vi "FindFocus.vi"(8 "error in (no error)":errorcluster, 11 "Transport":refnum<class "Transport.lvclass">) -> (0 "error out":errorcluster, 3 "Transport.lvclass":refnum<class "Transport.lvclass">)   [LabVIEW 2019, in "Transport.lvclass"]
uses:
  <userlib>/LevyLab/Transport/Transport/Transport.lvclass
  <userlib>/LevyLab/Transport/Control Experiment/Typedefs/Instruments--cluster.ctl
  <userlib>/LevyLab/Krohn Hite 7008/Instrument.KH7008.lvclass
  <userlib>/LevyLab/Lockin-Multichannel/Instrument.Lockin/Instrument.Lockin.lvclass
  <userlib>/LevyLab/Instrument Framework/Instrument Types/Cryostat/Instrument.Cryostat.lvclass
  <userlib>/LevyLab/Instrument Framework/Instrument Types/CBridge/Instrument.CBridge.lvclass
  <userlib>/LevyLab/Instrument Framework/Instrument Types/Delay Line/Instrument.DelayLine.lvclass
  <userlib>/LevyLab/Instrument Framework/Instrument Types/Strain/Instrument.Strain.lvclass
  <userlib>/LevyLab/Instrument Framework/Instrument Types/VNA/Instrument.VNA.lvclass
  <userlib>/LevyLab/Instrument Framework/Instrument Types/VSource/Instrument.VSource.lvclass
  <userlib>/LevyLab/Transport/Transport/Transport.lvclass/Transport.ctl
  <userlib>/LevyLab/Transport/Control Experiment/Control Experiment.lvclass/Control Experiment.ctl
  <userlib>/LevyLab/Lockin-Multichannel/Instrument.Lockin/Typedefs/Results Type--Enum.ctl
  <userlib>/LevyLab/Transport/Control Experiment/Control Experiment.lvclass
panel:
  in  "set \"Vsg\" to initial value?":bool
  in  "Tab Control":enum32{"LockIn Control", "Data", "Other"}(tab)
  out "elapsed time (s)":u32=1660
  in  "Input":i32[](array[numeric])=[21]
  in  "Vmax (end)":dbl=10.0 format="%#_3p"
  in  "Vmin (start)":dbl format="%#_3p"
  in  "dV":dbl=0.1 format="%#_3p"
  in  "Experiment Comments":string
  in  "Experiment Folder":string="Focus Optimization xxxxxxxx"
  out "T (mK)":dbl=0.001
  in  "wait after setting Control (ms)":u32=2000
  in  "Initial wait (ms)":u32=1000
  in  "Sweep":enum16{"Vsg", "Vbg", "Z-height", ""}(ring)=enum."Z-height"
  in  "cycles (1,2,...)":i32=1 min=1 step=1
  in  "phase":dbl
  out "Field (T)":dbl=-0.0003 format="%#_13g"
  in  "function (ramp)":enum16{"Ramp", "Triangle", "Sine"}(ring)
  out "time b/w points (ms)":u32=2066
  in  "stop":bool
  out "Mean vs. Parameter":cluster{dbl[], dbl[]}[](graph)
  out "X Lockins":cluster{dbl[], dbl[]}[](graph)
  out "Y Lockins":cluster{dbl[], dbl[]}[](graph)
  out "G4T":cluster{dbl[], dbl[]}[](graph)
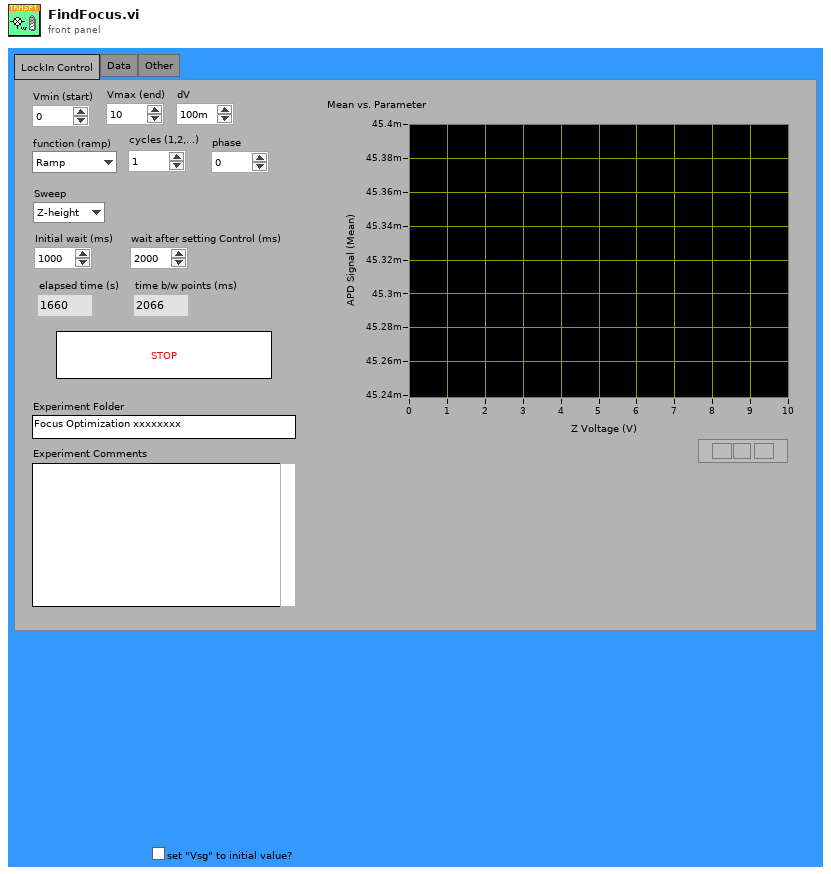
[diagram p1: front panel]
types:
  T1 = enum32{"Invalid", "Standard", "Closed", "Hidden", "Minimized", "Maximized"}
  T2 = enum32{"invalid app kind", "Development System", "Run Time System", "Student Edition", "Embedded LabVIEW", "Evaluation", "Custom"}
  T3 = typedef "Instrument.Lockin.lvclass/Results Type--Enum.ctl" = enum16{"X", "Y", "R", "Theta", "Mean"}
  T4 = typedef "Control Experiment.lvclass/Instruments--cluster.ctl" = cluster{"KH7008":refnum<class "Instrument.KH7008.lvclass">[], "Lockin":refnum<class "Instrument.Lockin.lvclass">, "Temperature":refnum<class "Instrument.Cryostat.lvclass">, "Magnet":refnum<class "Instrument.Cryostat.lvclass">, "Rotator":refnum<class "Instrument.Cryostat.lvclass">, "Level":refnum<class "Instrument.Cryostat.lvclass">, "Capacitance Bridge":refnum<class "Instrument.CBridge.lvclass">, "Delay Line":refnum<class "Instrument.DelayLine.lvclass">, "Strain Cell":refnum<class "Instrument.Strain.lvclass">, "VNA":refnum<class "Instrument.VNA.lvclass">, "Voltage Source":refnum<class "Instrument.VSource.lvclass">}
  T5 = cluster{"Core":cluster{"Current VI Reference":refnum<vi>, "Close Panel on Exit?":bool}, "Transport":refnum<class "Transport.lvclass">, "C.E.":refnum<class "Control Experiment.lvclass">, "Instruments":T4, "Sweep Values":dbl[], "Results (Dictionary)":cluster{"key":string, "value":dbl}[], "size":i32, "index":i32, "ms [0]":u32, "ms [i]":u32, "Execution:State":enum32{"Bad", "Idle", "Run top level", "Running"}}
  T6 = enum32{"Bad", "Idle", "Run top level", "Running"}
  T7 = cluster{"Current VI Reference":refnum<vi>, "Close Panel on Exit?":bool}
  T8 = cluster{"I-":i32, "I+":i32, "V1-":i32, "V1+":i32, "I2-":i32, "I2+":i32, "V2-":i32, "V2+":i32}
  T9 = typedef "Instrument.DAQ.lvclass/AO.Channel--Cluster--Array.ctl" = T10[]
  T10 = typedef "Instrument.DAQ.lvclass/AO.Channel--Cluster.ctl" = cluster{"Enable?":bool, "Channel":i32, "Amplitude":dbl, "Offset":dbl, "Frequency":dbl, "Phase":dbl, "Function":T11, "Sweeping?":bool}
  T11 = typedef "Instrument.DAQ.lvclass/AO.Channel.Function--Enum.ctl" = enum16{"Sine", "Triangle", "Square"}
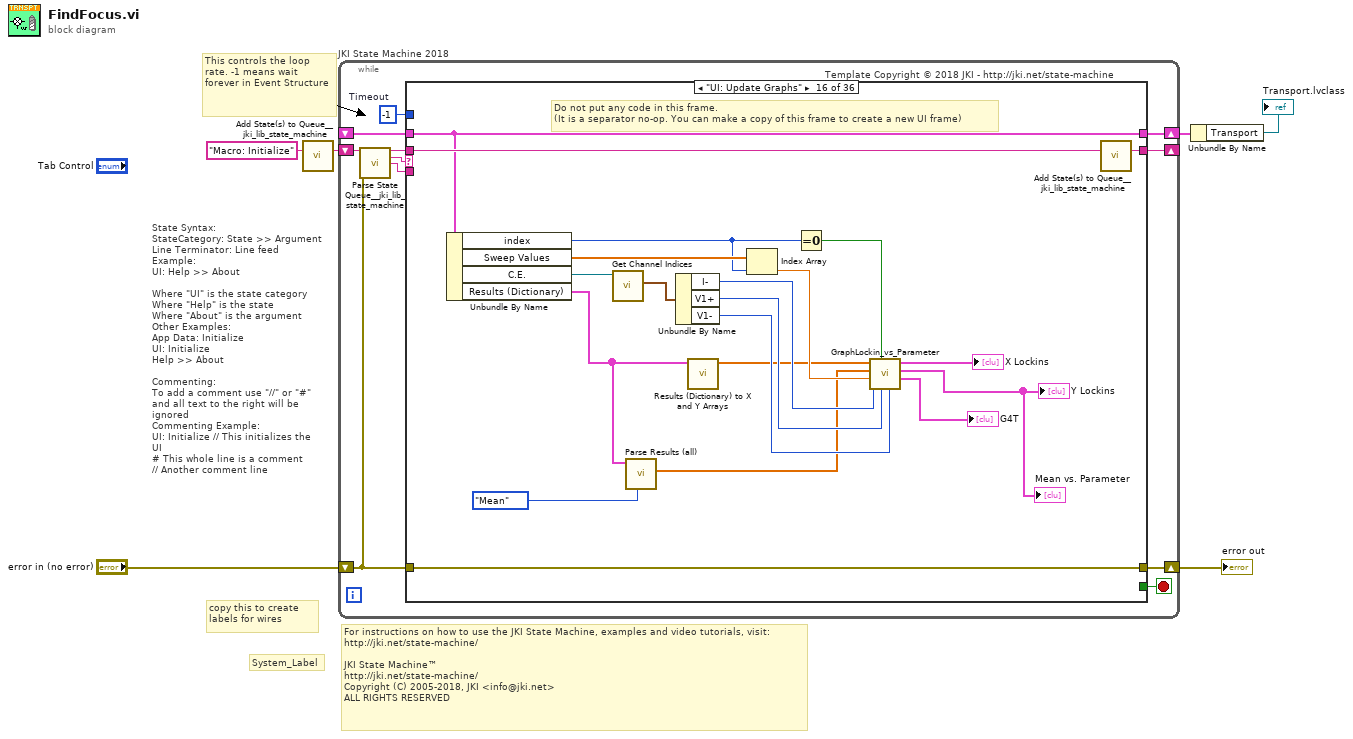
[diagram p0: block diagram]
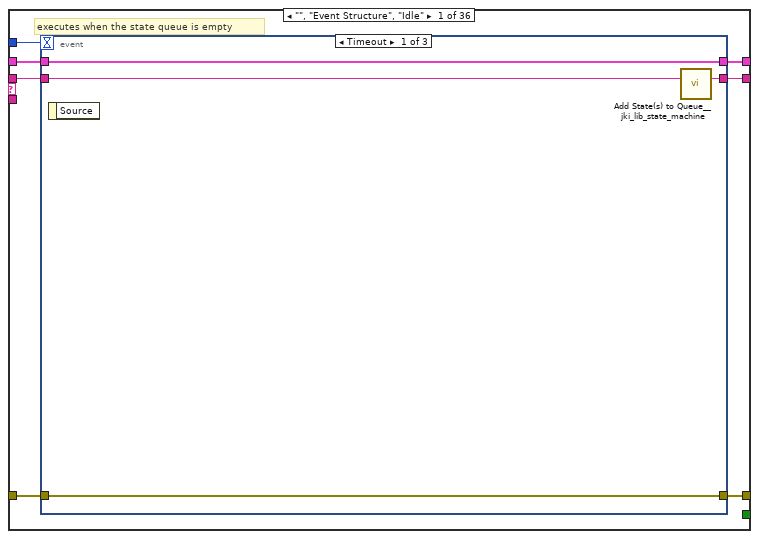
[diagram p2: hidden frame]
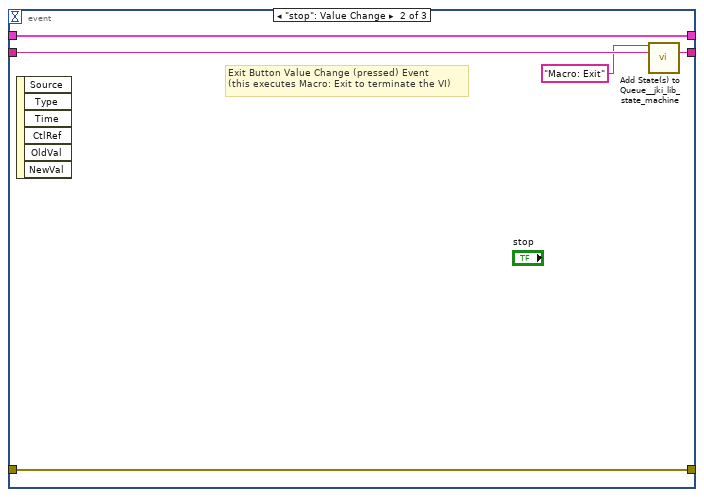
[diagram p3: hidden frame]
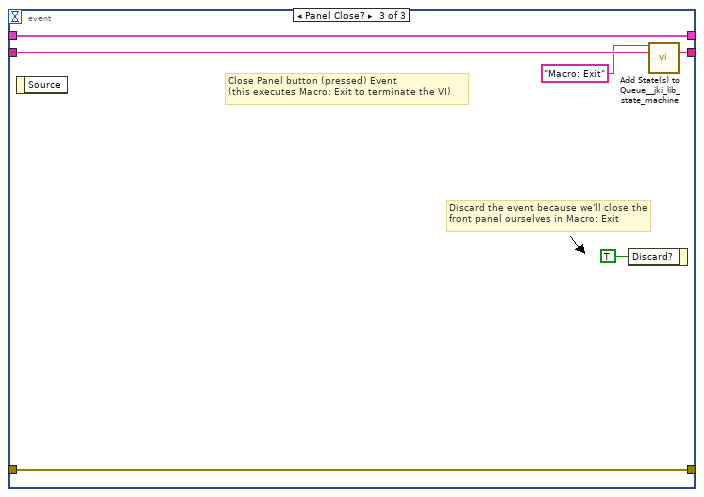
[diagram p4: hidden frame]
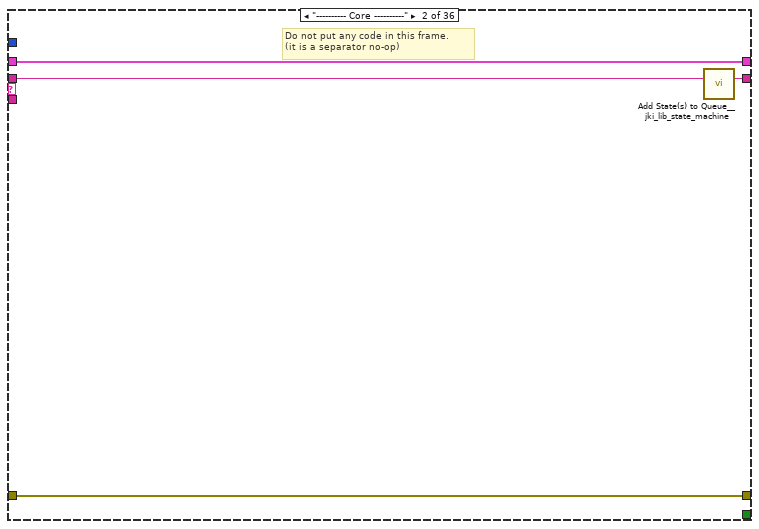
[diagram p5: hidden frame]
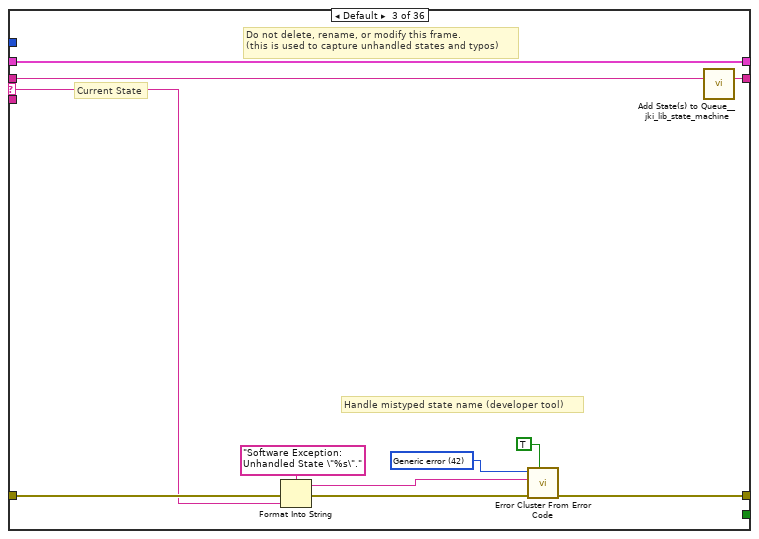
[diagram p6: hidden frame]
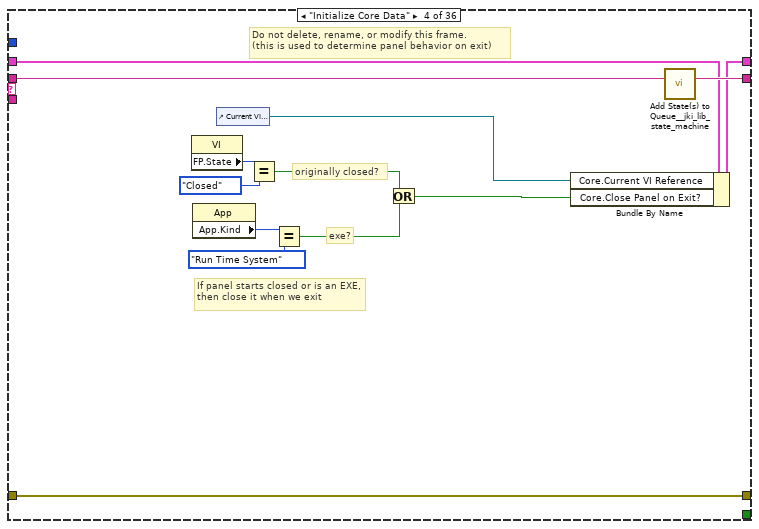
[diagram p7: hidden frame]
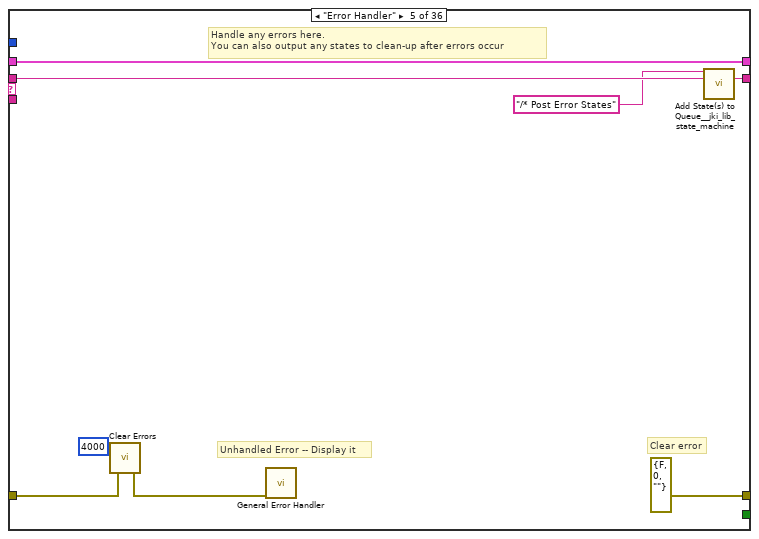
[diagram p8: hidden frame]
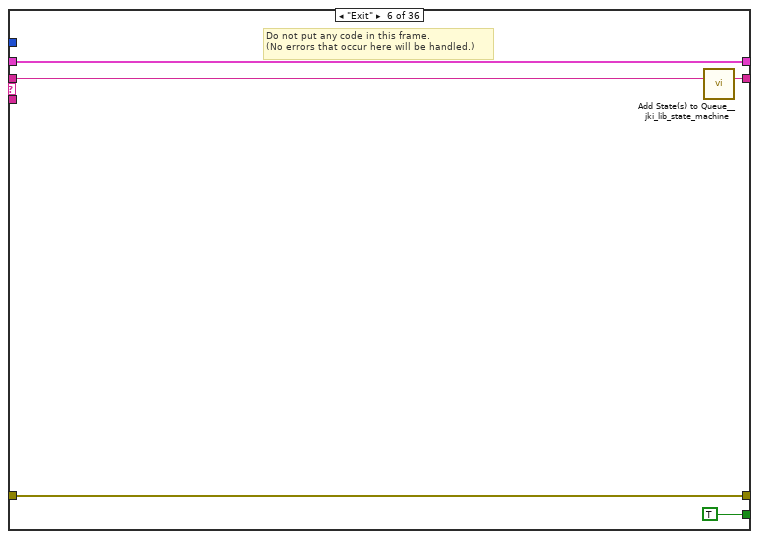
[diagram p9: hidden frame]
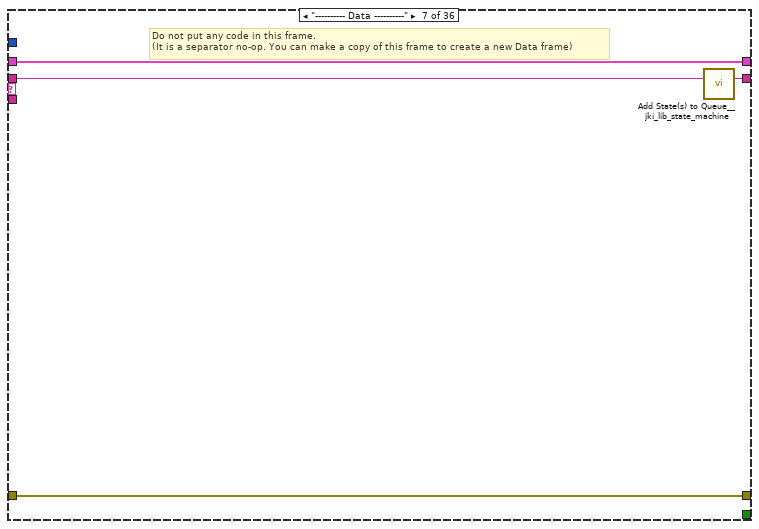
[diagram p10: hidden frame]
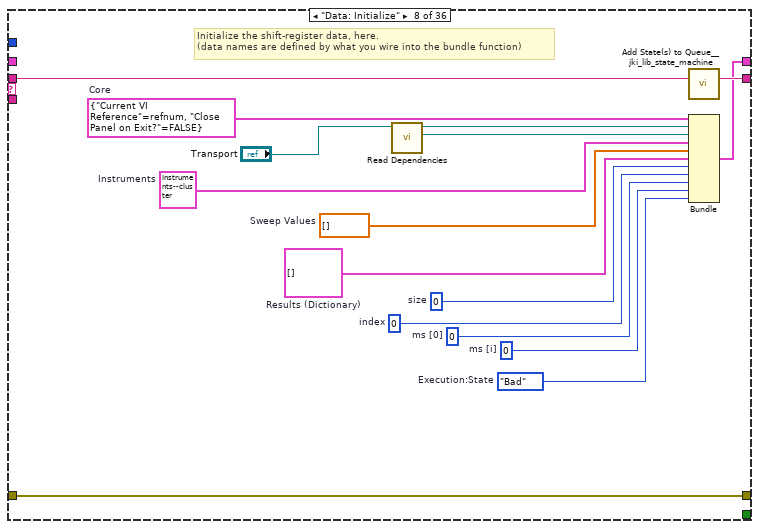
[diagram p11: hidden frame]
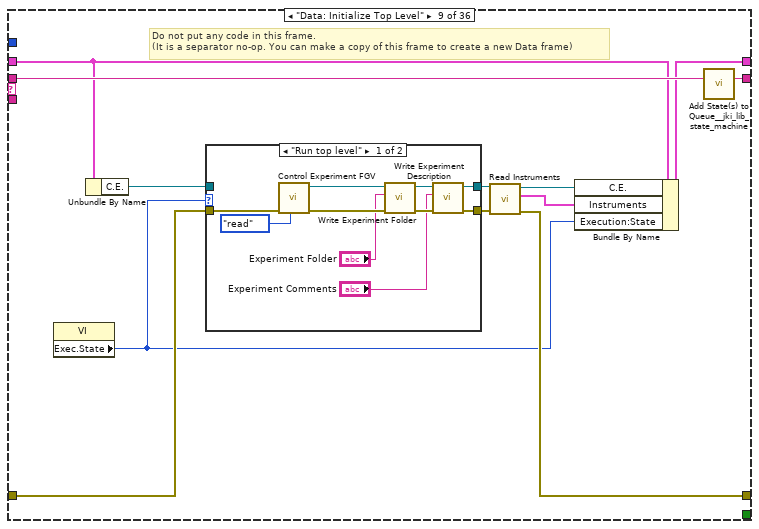
[diagram p12: hidden frame]
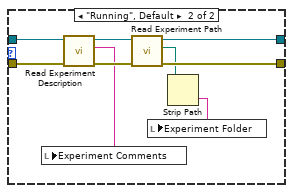
[diagram p13: hidden frame]
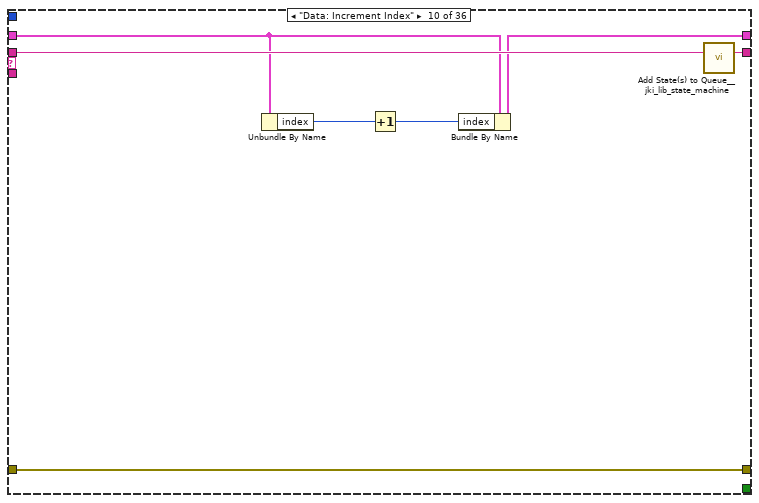
[diagram p14: hidden frame]
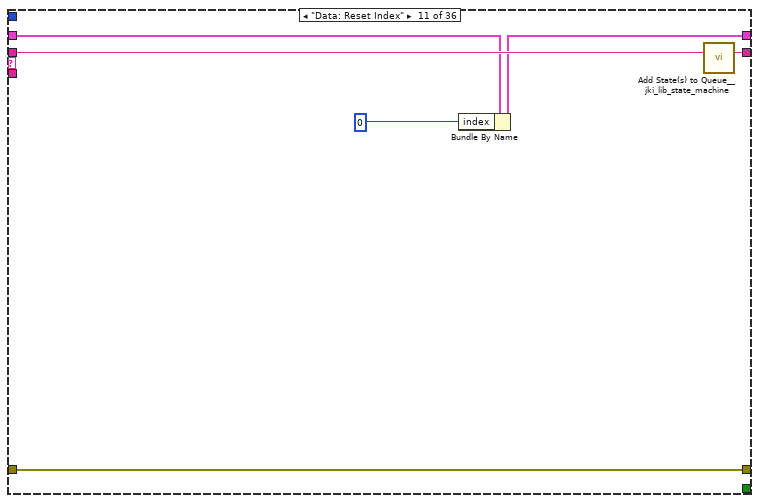
[diagram p15: hidden frame]
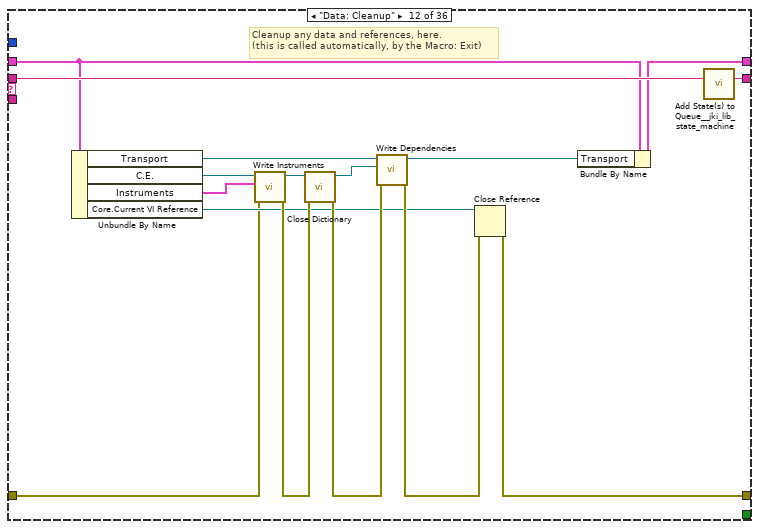
[diagram p16: hidden frame]
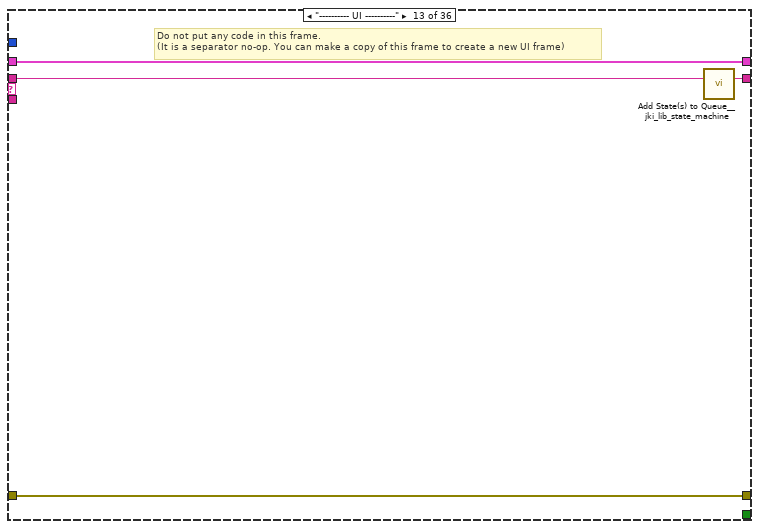
[diagram p17: hidden frame]
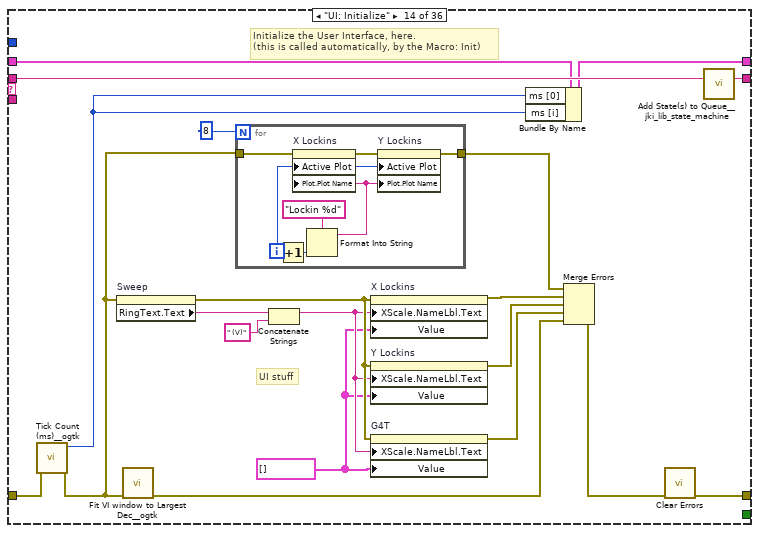
[diagram p18: hidden frame]
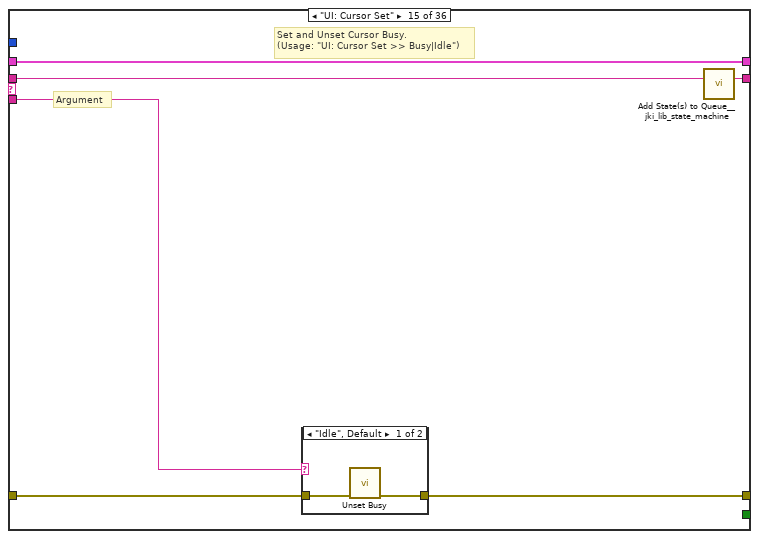
[diagram p19: hidden frame]
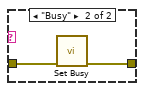
[diagram p20: hidden frame]
diagram:
  # "For instructions on how to use the JKI State Machine, examples and video tutorials, visit:\nhttp://jki.net/state-machine/\n\nJKI State Machine™\nhttp://jki.net/state-machine/\nCopyright (C) 2005-2018, JKI <info@jki.net>\nALL RIGHTS RESERVED"
  # "State Syntax:\nStateCategory: State >> Argument\nLine Terminator: Line feed\nExample:\nUI: Help >> About\n\nWhere \"UI\" is the state category\nWhere \"Help\" is the state\nWhere \"About\" is the argument\nOther Examples:\nApp Data: Initialize\nUI: Initialize\nHelp >> About\n\nCommenting:\nTo add a comment use \"//\" or \"#\" and all text to the right will be ignored\nCommenting Example:\nUI: Initialize // This initializes the UI\n# This whole line is a comment\n// Another comment line"
  # "copy this to create labels for wires"
  # "This controls the loop rate. -1 means wait forever in Event Structure"
  # "System_Label"
  n1 = call <vilib>:"Add State(s) to Queue__jki_lib_state_machine.vi"("State(s) in (\"\")"="Macro: Initialize") -> ("States Out"=w6:string)  [unwired: 14 in]
  n2 = while "JKI State Machine 2018" {
    shift-right: [w10] -> w4
    shift-left: _ -> [w9]
    shift-right: [w13] -> w2
    shift-left: "error in (no error)" -> [w7]
    shift-right: [w12] -> _
    shift-left: w6 -> [w14]
    stop <- w11 stop-if-true
    w8 = -1  # Timeout
    # "Template Copyright © 2018 JKI - http://jki.net/state-machine"
    n3 = call <vilib>:"Parse State Queue__jki_lib_state_machine.vi"("State Queue"=w14, "Error In (no error)"=w7) -> ("Remaining States"=w16:string, "Current State"=w17:string, "Arguments"=w15:string)  [unwired: 11 in]
    n4 = case shown="\"UI: Update Graphs\"" w17 {
      selector: w17 -> [_ _ w44 _ _ _ _ _ _ _ _ _ _ _ _ _ _ _ _ _ _ _ _ _ _ _ _ _ _ _ _ _ _ _ _ _]
      tunnel: w16 -> [w24 w43 w48 w67 w75 w80 w84 w100 w112 w138 w144 w160 w164 w184 w197 w221 w234 w241 w310 w315 w337 w347 w351 w375 w387 w394 w408 w463 w476 w489 w502 w520 w553 w557 w561 w571]
      tunnel: w15 -> [_ _ _ _ _ _ _ _ _ _ _ _ _ _ w192 _ _ w235 _ _ _ _ _ _ _ _ _ _ _ _ _ _ _ _ _ _]
      tunnel: w9 -> [w22 w40 w46 w60 w72 w78 w81 _ w103 w132 w141 w148 w161 w168 w195 w206 w229 w237 w307 w313 w330 w344 w348 w363 w384 w390 w398 w460 w472 w486 w497 w515 w549 w554 w558 w564]
      tunnel: [w21 w41 w50 w64 errorcluster {"status"=FALSE, "code"=0, "source"=""} ("error out") w77 w82 w97 w104 w136 w142 w145 w162 w173 w193 w219 w223 w238 w308 w311 w335 w345 w349 w353 w385 w391 w402 w461 w468 w480 w493 w511 w544 w555 w559 w568] -> w13
      tunnel: w7 -> [w20 w41 w49 w64 w69 w77 w82 w97 w105 w136 w142 w146 w162 w170 w194 w219 w231 w239 w308 w311 w335 w345 w349 w360 w385 w392 w401 w461 w473 w484 w494 w518 w545 w555 w559 w567]
      tunnel: [w23 w42 w47 w66 w74 w79 w83 w99 w111 w137 w143 w159 w163 w183 w196 w220 w233 w240 w309 w314 w336 w346 w350 w374 w386 w393 w407 w462 w475 w488 w501 w519 w552 w556 w560 w570] -> w12
      tunnel: [_ _ _ _ _ TRUE _ _ _ _ _ _ _ _ _ _ _ _ _ _ _ _ _ _ _ _ _ _ _ _ _ _ _ _ _ _] -> w11
      tunnel: [w19 w40 w46 w65 w72 w78 w81 w98 w102 w135 w140 w147 w161 w167 w195 w206 w228 w237 w307 w313 w330 w344 w348 w366 w384 w390 w399 w460 w471 w485 w496 w516 w550 w554 w558 w563] -> w10
      tunnel: w8 -> [w18 _ _ _ _ _ _ _ _ _ _ _ _ _ _ _ _ _ _ _ _ _ _ _ _ _ _ _ _ _ _ _ _ _ _ _]
      frame "", "Event Structure", "Idle" {
        # "executes when the state queue is empty"
        n5 = event shown="[0] Timeout" {
          selector: _ -> [_ _ _]
          dyn-events: _ -> [_ _ _]
          timeout: w18 -> [_ _ _]
          tunnel: w24 -> [w28 w33 w39]
          tunnel: [w27 w32 w38] -> w23
          tunnel: w22 -> [w25 w30 w36]
          tunnel: [w26 w31 w37] -> w21
          tunnel: w20 -> [w26 w31 w37]
          tunnel: [w25 w30 w36] -> w19
          event Timeout {
            n6 = event-data() -> ()  [unwired: 1 in, 1 out]
            n7 = call <vilib>:"Add State(s) to Queue__jki_lib_state_machine.vi"("State(s) in (\"\")"=w28) -> ("States Out"=w27:string)  [unwired: 14 in]
          }
          event "stop": Value Change {
            # "Exit Button Value Change (pressed) Event\n(this executes Macro: Exit to terminate the VI)"
            n8 = event-data() -> ()  [unwired: 1 in, 6 out]
            n9 = call <vilib>:"Add State(s) to Queue__jki_lib_state_machine.vi"("State(s) in Front (\"\")"="Macro: Exit", "State(s) in (\"\")"=w33) -> ("States Out"=w32:string)  [unwired: 13 in]
          }
          event Panel Close? {
            # "Discard the event because we'll close the front panel ourselves in Macro: Exit"
            # "Close Panel button (pressed) Event\n(this executes Macro: Exit to terminate the VI)"
            n10 = event-data() -> ()  [unwired: 1 in, 1 out]
            n11 = event-data("Discard?"=TRUE) -> ()  [unwired: 1 in, 1 out]
            n12 = call <vilib>:"Add State(s) to Queue__jki_lib_state_machine.vi"("State(s) in Front (\"\")"="Macro: Exit", "State(s) in (\"\")"=w39) -> ("States Out"=w38:string)  [unwired: 13 in]
          }
        }
      }
      frame "---------- Core ----------" {
        # "Do not put any code in this frame.\n(it is a separator no-op)"
        n13 = call <vilib>:"Add State(s) to Queue__jki_lib_state_machine.vi"("State(s) in (\"\")"=w43) -> ("States Out"=w42:string)  [unwired: 14 in]
      }
      frame Default {
        w53 = 42 items=["No error", "Argument error", "Memory is full", "Out of zone", "End of file", "File already open", "Generic file I/O error", "File not found", "File permission error", "Disk is full", "Duplicate path", "Too many files open", "System feature not enabled", "Resource file not found", "Cannot add resource", "Resource not found", "Image not found", "Image memory error", "Pen does not exist", "Config type invalid", "Config token not found", "Config parse error", "Config memory error", "Bad external code format", "Bad external code offset", "External code not present", "Null window", "Destroy window error", "Null menu", "Print aborted", "Bad print record", "Print driver error", "Windows error during printing", "Memory error during printing", "Print dialog error", "Generic print error", "Invalid device refnum", "Device not found", "Device parameter error", "Device unit error", "Cannot open device", "Device call aborted", "Generic error", "Cancelled by user", "Object ID too low", "Object ID too high", "Object not in heap", "Unknown heap", "Unknown object (invalid DefProc)", "Unknown object (DefProc not in table)", "Message out of range", "Invalid (null) method", "Unknown message", "Manager call not supported", "Bad address", "Network operation in progress", "Network operation timed out", "Connection is busy", "Network attribute not supported", "Network error", "Address in use", "System out of memory", "Connection aborted", "Connection refused", "Not connected", "Already connected", "Connection closed", "Initialization error (interapplication manager)", "Bad occurrence", "Wait on unbound occurrence handler", "Occurrence queue overflow", "Datalog type conflict", "Unused", "Unrecognized type (interapplication manager)", "Memory corrupt", "Failed to make temporary DLL", "Old CIN version", "Drag socket not found", "Failed to load drop-object", "Failed to register OLE object", "Failed to release OLE object", "Format specifier type mismatch", "Unknown format specifier", "Too few format specifiers", "Too many format specifiers", "Scan failed", "Newer CIN version", "Error converting to variant", "Runtime menu error", "Password tampered", "Variant attribute not found", "Incompatible variant data type", "Event data is not available", "Event Store is not present", "Occurrence is not found", "Event Queue is not created", "Event info is not available", "Refnum passed is NULL", "Error retrieving Class GUID", "Error retrieving CoClass GUID", "Error retrieving TypeLib GUID.", "Bad built application magic bytes.", "Specific driver is different from the specific driver associated with the Logical Name.", "There is no session opened to the class driver.", "Max Error", "MAX - Error with config objects", "MAX - Error loading configuration", "MAX - Group not supported"]
        # "Current State"
        # "Do not delete, rename, or modify this frame.\n(this is used to capture unhandled states and typos)"
        # "Handle mistyped state name (developer tool)"
        n14 = Format Into String(format string="Software Exception: Unhandled State \"%s\"." ("message"), error in=w49, w44) -> (resulting string=w52:string, error out=w51:errorcluster)  [unwired: 1 in]
        n15 = call <vilib>:"Error Cluster From Error Code.vi"("show call chain? (False)"=TRUE, "error in (no error)"=w51, "error message (\"\")"=w52, "error code (0)"=w53) -> ("error out"=w50:errorcluster)  [unwired: 5 in]
        n16 = call <vilib>:"Add State(s) to Queue__jki_lib_state_machine.vi"("State(s) in (\"\")"=w48) -> ("States Out"=w47:string)  [unwired: 14 in]
      }
      frame "Initialize Core Data" {
        # "Do not delete, rename, or modify this frame.\n(this is used to determine panel behavior on exit)"
        # "originally closed?"
        # "exe?"
        # "If panel starts closed or is an EXE, then close it when we exit"
        n17 = property class="VI"() -> ("FP.State"=w57:T1)  [unwired: 2 in, 2 out]
        n18 = property class="App"() -> ("App.Kind"=w63:T2)  [unwired: 2 in, 2 out]
        n19 = control-ref of="Current VI Reference"() -> (w58:refnum<vi>)
        n20 = Equal?(x=w57, y=T1."Closed" ("Front Panel Window:State")) -> (x = y?=w55:bool)
        n21 = Equal?(x=w63, y=T2."Run Time System" ("Application:Kind")) -> (x = y?=w61:bool)
        n22 = Or(x=w55, y=w61) -> (x .or. y?=w59:bool)
        n23 = Bundle By Name(cluster=w60, "Core.Current VI Reference"=w58, "Core.Close Panel on Exit?"=w59) -> (w65:T5)
        n24 = call <vilib>:"Add State(s) to Queue__jki_lib_state_machine.vi"("State(s) in (\"\")"=w67) -> ("States Out"=w66:string)  [unwired: 14 in]
      }
      frame "Error Handler" {
        # "Unhandled Error -- Display it"
        # "Handle any errors here.\nYou can also output any states to clean-up after errors occur"
        # "Clear error"
        n25 = call <vilib>:"Clear Errors.vi"("error in (no error)"=w69, "specific error code to clear (0: all)"=4000) -> ("error out"=w68:errorcluster)  [unwired: 4 in, 1 out]
        n26 = call <vilib>:"General Error Handler.vi"("error in (no error)"=w68) -> ()  [unwired: 10 in, 5 out]
        n27 = call <vilib>:"Add State(s) to Queue__jki_lib_state_machine.vi"("State(s) in Front (\"\")"="/* Post Error States", "State(s) in (\"\")"=w75) -> ("States Out"=w74:string)  [unwired: 13 in]
      }
      frame "Exit" {
        # "Do not put any code in this frame.\n(No errors that occur here will be handled.)"
        n28 = call <vilib>:"Add State(s) to Queue__jki_lib_state_machine.vi"("State(s) in (\"\")"=w80) -> ("States Out"=w79:string)  [unwired: 14 in]
      }
      frame "---------- Data ----------" {
        # "Do not put any code in this frame.\n(It is a separator no-op. You can make a copy of this frame to create a new Data frame)"
        n29 = call <vilib>:"Add State(s) to Queue__jki_lib_state_machine.vi"("State(s) in (\"\")"=w84) -> ("States Out"=w83:string)  [unwired: 14 in]
      }
      frame "Data: Initialize" {
        w85 = cluster{"key":string, "value":dbl}[] []  # Results (Dictionary)
        w89 = T6."Bad"  # Execution:State
        w90 = 0  # size
        w91 = u32 0  # ms [i]
        w92 = u32 0  # ms [0]
        w93 = 0  # index
        w94 = dbl[] []  # Sweep Values
        w95 = T4 {"KH7008"=[], "Lockin"=refnum, "Temperature"=refnum, "Magnet"=refnum, "Rotator"=refnum, "Level"=refnum, "Capacitance Bridge"=refnum, "Delay Line"=refnum, "Strain Cell"=refnum, "VNA"=refnum, "Voltage Source"=refnum}  # Instruments
        w96 = T7 {"Current VI Reference"=refnum, "Close Panel on Exit?"=FALSE}  # Core
        # "Initialize the shift-register data, here.\n(data names are defined by what you wire into the bundle function)"
        n30 = call <userlib>:"Read Dependencies.vi"("Transport"="Transport") -> ("C.E."=w87:refnum<class "Control Experiment.lvclass">, "Transport"=w86:refnum<class "Transport.lvclass">)  [unwired: 8 in, 1 out]
        n31 = call <vilib>:"Add State(s) to Queue__jki_lib_state_machine.vi"("State(s) in (\"\")"=w100) -> ("States Out"=w99:string)  [unwired: 14 in]
        n32 = Bundle("Core"=w96, "Transport"=w86, "C.E."=w87, "Instruments"=w95, "Sweep Values"=w94, "Results (Dictionary)"=w85, "size"=w90, "index"=w93, "ms [0]"=w92, "ms [i]"=w91, "Execution:State"=w89) -> (w98:T5)  [unwired: 1 in]
      }
      frame "Data: Initialize Top Level" {
        # "Do not put any code in this frame.\n(It is a separator no-op. You can make a copy of this frame to create a new Data frame)"
        n33 = property class="VI"() -> ("Exec.State"=w101:T6)  [unwired: 2 in, 2 out]
        n34 = Unbundle By Name(w103) -> ("C.E."=w106:refnum<class "Control Experiment.lvclass">)
        n35 = case shown="\"Run top level\"" w101 {
          tunnel: w105 -> [w122 w130]
          tunnel: [w117 w126] -> w107
          tunnel: [w116 w127] -> w108
          tunnel: w106 -> [_ w131]
          frame "Run top level" {
            n36 = call <userlib>:"Control Experiment FGV.vi"("Function"=enum16{"read", "write"}."read", "error in (no error)"=w122) -> ("error out"=w120:errorcluster, "Control Experiment.lvclass out"=w121:refnum<class "Control Experiment.lvclass">)  [unwired: 8 in]
            n37 = call <userlib>:"Write Experiment Folder.vi"("error in (no error)"=w120, "Experiment Folder"="Experiment Folder", "Control Experiment in"=w121) -> ("error out"=w118:errorcluster, "Control Experiment out"=w119:refnum<class "Control Experiment.lvclass">)  [unwired: 7 in]
            n38 = call <userlib>:"Write Experiment Description.vi"("error in (no error)"=w118, "Experiment Description"="Experiment Comments", "Control Experiment in"=w119) -> ("error out"=w117:errorcluster, "Control Experiment out"=w116:refnum<class "Control Experiment.lvclass">)  [unwired: 7 in]
          }
          frame "Running", Default {
            n39 = call <userlib>:"Read Experiment Description.vi"("error in (no error)"=w130, "Control Experiment in"=w131) -> ("error out"=w129:errorcluster, "Experiment Description"=w124:string, "Control Experiment out"=w128:refnum<class "Control Experiment.lvclass">)  [unwired: 7 in]
            n40 = local write "Experiment Comments"(w124) -> ()
            n41 = call <userlib>:"Read Experiment Path.vi"("error in (no error)"=w129, "Control Experiment in"=w128) -> ("error out"=w126:errorcluster, "Experiment Path"=w125:path, "Control Experiment out"=w127:refnum<class "Control Experiment.lvclass">)  [unwired: 7 in]
            n42 = Strip Path(path=w125) -> (name=w123:string)  [unwired: 1 out]
            n43 = local write "Experiment Folder"(w123) -> ()
          }
        }
        n44 = call <userlib>:"Read Instruments.vi"("error in (no error)"=w107, "Control Experiment in"=w108) -> ("error out"=w104:errorcluster, "Instruments"=w110:T4, "Control Experiment out"=w109:refnum<class "Control Experiment.lvclass">)  [unwired: 7 in]
        n45 = Bundle By Name(cluster=w103, "C.E."=w109, "Instruments"=w110, "Execution:State"=w101) -> (w102:T5)
        n46 = call <vilib>:"Add State(s) to Queue__jki_lib_state_machine.vi"("State(s) in (\"\")"=w112) -> ("States Out"=w111:string)  [unwired: 14 in]
      }
      frame "Data: Increment Index" {
        n47 = Unbundle By Name(w132) -> ("index"=w134:i32)
        n48 = Increment(x=w134) -> (x+1=w133:i32)
        n49 = Bundle By Name(cluster=w132, "index"=w133) -> (w135:T5)
        n50 = call <vilib>:"Add State(s) to Queue__jki_lib_state_machine.vi"("State(s) in (\"\")"=w138) -> ("States Out"=w137:string)  [unwired: 14 in]
      }
      frame "Data: Reset Index" {
        n51 = Bundle By Name(cluster=w141, "index"=0) -> (w140:T5)
        n52 = call <vilib>:"Add State(s) to Queue__jki_lib_state_machine.vi"("State(s) in (\"\")"=w144) -> ("States Out"=w143:string)  [unwired: 14 in]
      }
      frame "Data: Cleanup" {
        # "Cleanup any data and references, here.\n(this is called automatically, by the Macro: Exit)"
        n53 = Unbundle By Name(w148) -> ("Transport"=w157:refnum<class "Transport.lvclass">, "C.E."=w155:refnum<class "Control Experiment.lvclass">, "Instruments"=w153:T4, "Core.Current VI Reference"=w149:refnum<vi>)
        n54 = call <userlib>:"Write Instruments.vi"("error in (no error)"=w146, "Instruments"=w153, "Control Experiment in"=w155) -> ("error out"=w152:errorcluster, "Control Experiment out"=w154:refnum<class "Control Experiment.lvclass">)  [unwired: 7 in]
        n55 = call <userlib>:"Close Dictionary.vi"("error in (no error)"=w152, "Control Experiment in"=w154) -> ("error out"=w151:errorcluster, "Control Experiment out"=w156:refnum<class "Control Experiment.lvclass">)  [unwired: 8 in]
        n56 = call <userlib>:"Write Dependencies.vi"("error in (no error)"=w151, "Control Experiment"=w156, "Transport in"=w157) -> ("error out"=w150:errorcluster, "Transport out"=w158:refnum<class "Transport.lvclass">)  [unwired: 7 in]
        n57 = Close Reference(reference=w149, error in (no error)=w150) -> (error out=w145:errorcluster)
        n58 = Bundle By Name(cluster=w148, "Transport"=w158) -> (w147:T5)
        n59 = call <vilib>:"Add State(s) to Queue__jki_lib_state_machine.vi"("State(s) in (\"\")"=w160) -> ("States Out"=w159:string)  [unwired: 14 in]
      }
      frame "---------- UI ----------" {
        # "Do not put any code in this frame.\n(It is a separator no-op. You can make a copy of this frame to create a new UI frame)"
        n60 = call <vilib>:"Add State(s) to Queue__jki_lib_state_machine.vi"("State(s) in (\"\")"=w164) -> ("States Out"=w163:string)  [unwired: 14 in]
      }
      frame "UI: Initialize" {
        w165 = cluster{dbl[], dbl[]}[] [] ("G4T")
        # "UI stuff"
        # "Initialize the User Interface, here.\n(this is called automatically, by the Macro: Init)"
        n61 = call <userlib>:"Tick Count (ms)__ogtk.vi"("error in (no error)"=w170) -> ("error out"=w169:errorcluster, "millisecond timer value"=w166:u32)  [unwired: 9 in]
        n62 = property on="Sweep" class="Enum (strict)"(error in=w169) -> (error out=w178:errorcluster, "RingText.Text"=w176:string)  [unwired: 1 in, 1 out]
        n63 = call <userlib>:"Fit VI window to Largest Dec__ogtk.vi"("error in (no error)"=w169) -> ("error out"=w172:errorcluster)  [unwired: 5 in, 1 out]
        n64 = for {
          N: 8 -> [_]
          tunnel: [w185] -> w179
          tunnel: w169 -> [w190]
          i -> [w188]
          n65 = Increment(x=w188) -> (x+1=w186:i32)
          n66 = Format Into String(format string="Lockin %d", w186) -> (resulting string=w189:string)  [unwired: 2 in, 1 out]
          n67 = property on="X Lockins" class="XYGraph (strict)"(error in=w190, "Active Plot"=w188, "Plot.Plot Name"=w189) -> (error out=w187:errorcluster)  [unwired: 1 in, 1 out]
          n68 = property on="Y Lockins" class="XYGraph (strict)"(error in=w187, "Active Plot"=w188, "Plot.Plot Name"=w189) -> (error out=w185:errorcluster)  [unwired: 1 in, 1 out]
        }
        n69 = Concatenate Strings(w176, " (V)" ("string")) -> (w177:string)
        n70 = property on="X Lockins" class="XYGraph (strict)"(error in=w178, "XScale.NameLbl.Text"=w177, "Value"=w165) -> (error out=w180:errorcluster)  [unwired: 1 in, 1 out]
        n71 = property on="Y Lockins" class="XYGraph (strict)"(error in=w178, "XScale.NameLbl.Text"=w177, "Value"=w165) -> (error out=w181:errorcluster)  [unwired: 1 in, 1 out]
        n72 = property on="G4T" class="XYGraph (strict)"(error in=w178, "XScale.NameLbl.Text"=w177, "Value"=w165) -> (error out=w182:errorcluster)  [unwired: 1 in, 1 out]
        n73 = Bundle By Name(cluster=w168, "ms [0]"=w166, "ms [i]"=w166) -> (w167:T5)
        n74 = Merge Errors(w179, w180, w181, w182, w172) -> (w171:errorcluster)
        n75 = call <vilib>:"Clear Errors.vi"("error in (no error)"=w171) -> ("error out"=w173:errorcluster)  [unwired: 5 in, 1 out]
        n76 = call <vilib>:"Add State(s) to Queue__jki_lib_state_machine.vi"("State(s) in (\"\")"=w184) -> ("States Out"=w183:string)  [unwired: 14 in]
      }
      frame "UI: Cursor Set" {
        # "Argument"
        # "Set and Unset Cursor Busy.\n(Usage: \"UI: Cursor Set >> Busy|Idle\")"
        n77 = case shown="\"Idle\", Default" w192 {
          tunnel: w194 -> [w199 w201]
          tunnel: [w198 w200] -> w193
          frame "Idle", Default {
            n78 = call <vilib>:"Unset Busy.vi"("error in (no error)"=w199) -> ("error out"=w198:errorcluster)  [unwired: 10 in]
          }
          frame "Busy" {
            n79 = call <vilib>:"Set Busy.vi"("error in (no error)"=w201) -> ("error out"=w200:errorcluster)  [unwired: 9 in, 1 out]
          }
        }
        n80 = call <vilib>:"Add State(s) to Queue__jki_lib_state_machine.vi"("State(s) in (\"\")"=w197) -> ("States Out"=w196:string)  [unwired: 14 in]
      }
      frame "UI: Update Graphs" {
        # "Do not put any code in this frame.\n(It is a separator no-op. You can make a copy of this frame to create a new UI frame)"
        n81 = Unbundle By Name(w206) -> ("index"=w208:i32, "Sweep Values"=w211:dbl[], "C.E."=w217:refnum<class "Control Experiment.lvclass">, "Results (Dictionary)"=w205:cluster{"key":string, "value":dbl}[])
        n82 = call <userlib>:"Get Channel Indices.vi"("Control Experiment in"=w217) -> ("Indices"=w216:T8)  [unwired: 8 in, 2 out]
        n83 = call <userlib>:"Parse Results (all).vi"("Type"=Results_Type--Enum."Mean", "Results (Dictionary)"=w205) -> ("Data"=w203:dbl[])  [unwired: 6 in, 3 out]
        n84 = Unbundle By Name(w216) -> ("I-"=w213:i32, "V1+"=w215:i32, "V1-"=w214:i32)
        n85 = call <userlib>:"Results (Dictionary) to X and Y Arrays.vi"("Results (Dictionary)"=w205) -> ("X"=w207:dbl[])  [unwired: 9 in, 1 out]
        n86 = Index Array(array=w211, index=w208) -> (element=w210:dbl)
        n87 = Equal To 0?(x=w208) -> (x = 0?=w209:bool)
        n88 = call <userlib>:"GraphLockin_vs_Parameter.vi"("V-"=w214, "V+"=w215, "reset?"=w209, "Current"=w213, "Parameter"=w210, "Y[ ]"=w203, "X[ ]"=w207) -> ("G(e2/h) vs Parameter"=→"G4T":cluster{"Y":dbl[], "Y":dbl[]}[], "Y vs Parameter"=→"Y Lockins" →"Mean vs. Parameter":cluster{dbl[], dbl[]}[], "X vs Parameter"=→"X Lockins":cluster{dbl[], dbl[]}[])  [unwired: 1 in, 1 out]
        n89 = call <vilib>:"Add State(s) to Queue__jki_lib_state_machine.vi"("State(s) in (\"\")"=w221) -> ("States Out"=w220:string)  [unwired: 14 in]
      }
      frame "UI: Update Timer" {
        n90 = Unbundle By Name(w229) -> ("ms [0]"=w230:u32)
        n91 = call <userlib>:"Tick Count (ms)__ogtk.vi"("error in (no error)"=w231) -> ("error out"=w224:errorcluster, "millisecond timer value"=w222:u32)  [unwired: 9 in]
        n92 = Subtract(x=w222, y=w230) -> (x-y=w226:u32)
        n93 = call <userlib>:"MGI Milliseconds Since Last Call.vi"("Error In"=w224) -> ("ms"=→"time b/w points (ms)":u32, "Error Out"=w223:errorcluster)  [unwired: 5 in]
        n94 = Divide(x=w226, y=u32 1000 ("x")) -> (x/y=→"elapsed time (s)":dbl)
        n95 = Bundle By Name(cluster=w229, "ms [i]"=w222) -> (w228:T5)
        n96 = call <vilib>:"Add State(s) to Queue__jki_lib_state_machine.vi"("State(s) in (\"\")"=w234) -> ("States Out"=w233:string)  [unwired: 14 in]
      }
      frame "UI: Front Panel State" {
        # "Argument"
        # "Set Front Panel Open or Closed\n(Usage: \"UI: Front Panel State >> Open|Close\")"
        n97 = Unbundle By Name(w237) -> ("Core.Current VI Reference"=w236:refnum<vi>)
        n98 = case shown="\"Minimize\", \"Minimized\"" w235 {
          tunnel: w239 -> [w247 w262 w273 w286 w299]
          tunnel: [w249 w263 w275 w288 w301] -> w238
          tunnel: w236 -> [w248 w260 w274 w287 w300]
          frame "Open", "Standard", Default {
            w242 = T1."Standard" ("State")
            n99 = property class="VI"(reference=w248, error in=w247) -> (reference out=w245:refnum<vi>, error out=w246:errorcluster, "FP.State"=w244:T1)
            n100 = Not Equal?(x=w244, y=w242) -> (x != y?=w243:bool)
            n101 = case shown="True" w243 {
              tunnel: [w253 w255] -> w249
              tunnel: w246 -> [w252 w255]
              tunnel: w245 -> [w251 _]
              tunnel: w242 -> [w250 _]
              frame True {
                n102 = invoke class="VI" method="FP.Open"(reference=w251, error in=w252, "Activate"=TRUE, "State"=w250) -> (error out=w253:errorcluster)  [unwired: 1 in, 4 out]
              }
              frame False {
              }
            }
          }
          frame "Close", "Closed" {
            n103 = property class="VI"(reference=w260, error in=w262) -> (reference out=w259:refnum<vi>, error out=w261:errorcluster, "FP.State"=w257:T1)
            n104 = Not Equal?(x=w257, y=T1."Closed" ("Front Panel Window:State")) -> (x != y?=w256:bool)
            n105 = case shown="True" w256 {
              tunnel: [w264 w267] -> w263
              tunnel: w261 -> [w264 w266]
              tunnel: w259 -> [_ w265]
              frame False {
              }
              frame True {
                n106 = invoke class="VI" method="FP.Close"(reference=w265, error in=w266) -> (error out=w267:errorcluster)  [unwired: 1 in, 2 out]
              }
            }
          }
          frame "Hidden", "Hide" {
            w268 = T1."Hidden" ("State")
            n107 = property class="VI"(reference=w274, error in=w273) -> (reference out=w271:refnum<vi>, error out=w272:errorcluster, "FP.State"=w270:T1)
            n108 = Not Equal?(x=w270, y=w268) -> (x != y?=w269:bool)
            n109 = case shown="True" w269 {
              tunnel: [w279 w280] -> w275
              tunnel: w272 -> [w278 w280]
              tunnel: w271 -> [w277 _]
              tunnel: w268 -> [w276 _]
              frame True {
                n110 = invoke class="VI" method="FP.Open"(reference=w277, error in=w278, "State"=w276) -> (error out=w279:errorcluster)  [unwired: 2 in, 4 out]
              }
              frame False {
              }
            }
          }
          frame "Minimize", "Minimized" {
            w281 = T1."Minimized" ("State")
            n111 = property class="VI"(reference=w287, error in=w286) -> (reference out=w284:refnum<vi>, error out=w285:errorcluster, "FP.State"=w283:T1)
            n112 = Not Equal?(x=w283, y=w281) -> (x != y?=w282:bool)
            n113 = case shown="True" w282 {
              tunnel: [w292 w293] -> w288
              tunnel: w285 -> [w291 w293]
              tunnel: w284 -> [w290 _]
              tunnel: w281 -> [w289 _]
              frame True {
                n114 = invoke class="VI" method="FP.Open"(reference=w290, error in=w291, "State"=w289) -> (error out=w292:errorcluster)  [unwired: 2 in, 4 out]
              }
              frame False {
              }
            }
          }
          frame "Maximize", "Maximized" {
            w294 = T1."Maximized" ("State")
            n115 = property class="VI"(reference=w300, error in=w299) -> (reference out=w297:refnum<vi>, error out=w298:errorcluster, "FP.State"=w296:T1)
            n116 = Not Equal?(x=w296, y=w294) -> (x != y?=w295:bool)
            n117 = case shown="True" w295 {
              tunnel: [w305 w306] -> w301
              tunnel: w298 -> [w304 w306]
              tunnel: w297 -> [w303 _]
              tunnel: w294 -> [w302 _]
              frame True {
                n118 = invoke class="VI" method="FP.Open"(reference=w303, error in=w304, "State"=w302) -> (error out=w305:errorcluster)  [unwired: 2 in, 4 out]
              }
              frame False {
              }
            }
          }
        }
        n119 = call <vilib>:"Add State(s) to Queue__jki_lib_state_machine.vi"("State(s) in (\"\")"=w241) -> ("States Out"=w240:string)  [unwired: 14 in]
      }
      frame "---------- Macro ----------" {
        # "Do not put any code in this frame.\n(It is a separator no-op. You can make a copy of this frame to create a new Macro frame)"
        n120 = call <vilib>:"Add State(s) to Queue__jki_lib_state_machine.vi"("State(s) in (\"\")"=w310) -> ("States Out"=w309:string)  [unwired: 14 in]
      }
      frame "Macro: Initialize" {
        # "Initialization Macro\n(This is called once, when the VI starts)"
        n121 = call <vilib>:"Add State(s) to Queue__jki_lib_state_machine.vi"("State(s) in Front (\"\")"="Data: Initialize\nInitialize Core Data\nUI: Initialize\nUI: Front Panel State >> Open\nData: Initialize Top Level\nData: Reset Index\nMeasure: Temperature\nMeasure: Magnet\nMeasure: Capacitance\nSweep: Initialize\nMacro: Sweep", "State(s) in (\"\")"=w315) -> ("States Out"=w314:string)  [unwired: 13 in]
      }
      frame "Macro: Sweep" {
        # "stop if true"
        # "continue if true"
        # "sweep is finished"
        # "keep sweeping"
        # "Do not put any code in this frame.\n(It is a separator no-op. You can make a copy of this frame to create a new Macro frame)"
        n122 = Unbundle By Name(w330) -> ("size"=w331:i32, "index"=w334:i32)
        n123 = Decrement(x=w331) -> (x-1=w324:i32)
        n124 = local read "stop"() -> (w317:bool)
        n125 = Not Equal?(x=w324, y=w334) -> (x != y?=w319:bool)
        n126 = Not(x=w317) -> (.not. x?=w318:bool)
        n127 = And(x=w318, y=w319) -> (x .and. y?=w316:bool)
        n128 = Select(t="Data: Reset Index\nConfigure: Set" ("State(s) in Front (\"\")"), s="set \"Vsg\" to initial value?", f="" ("State(s) in Front (\"\")")) -> (s? t:f=w321:string)
        n129 = call <vilib>:"Add State(s) to Queue__jki_lib_state_machine.vi"("State(s) in Front (\"\")"="File: Save" ("State(s) in Front (\"\")"), "State(s) in (\"\")"=w321, "State(s) at Back (\"\")"="Macro: Exit" ("State(s) in Front (\"\")")) -> ("States Out"=w325:string)  [unwired: 12 in]
        n130 = Select(t="Macro: Sweep" ("State(s) in Front (\"\")"), s=w316, f=w325) -> (s? t:f=w333:string)
        n131 = call <vilib>:"Add State(s) to Queue__jki_lib_state_machine.vi"("State(s) in Front (\"\")"="Configure: Set\nConfigure: Wait\nMeasure: Lockin\nMeasure: Time\n//Measure: Temperature\nUI: Update Graphs\nUI: Update Timer\nData: Increment Index" ("State(s) in Front (\"\")"), "State(s) at Back (\"\")"=w333) -> ("States Out"=w323:string)  [unwired: 13 in]
        n132 = call <vilib>:"Add State(s) to Queue__jki_lib_state_machine.vi"("State(s) in (\"\")"=w337, "State(s) at Back (\"\")"=w323) -> ("States Out"=w336:string)  [unwired: 13 in]
      }
      frame "Macro: Exit" {
        # "Exit Macro\n(This is called once, when the VI exits)"
        n133 = Unbundle By Name(w344) -> ("Core.Close Panel on Exit?"=w343:bool)
        n134 = Select(t="UI: Front Panel State >> Close", s=w343, f="") -> (s? t:f=w340:string)
        n135 = call <vilib>:"Add State(s) to Queue__jki_lib_state_machine.vi"("State(s) in (\"\")"=w340, "State(s) at Back (\"\")"="Data: Cleanup\nExit") -> ("States Out"=w338:string)  [unwired: 13 in]
        n136 = call <vilib>:"Add State(s) to Queue__jki_lib_state_machine.vi"("State(s) in Front (\"\")"=w338, "State(s) in (\"\")"=w347) -> ("States Out"=w346:string)  [unwired: 13 in]
      }
      frame "---------- Sweep ----------" {
        # "Do not put any code in this frame.\n(It is a separator no-op. You can make a copy of this frame to create a new Macro frame)"
        n137 = call <vilib>:"Add State(s) to Queue__jki_lib_state_machine.vi"("State(s) in (\"\")"=w351) -> ("States Out"=w350:string)  [unwired: 14 in]
      }
      frame "Sweep: Initialize" {
        # "define sweep"
        # "Do not put any code in this frame.\n(It is a separator no-op. You can make a copy of this frame to create a new Macro frame)"
        n138 = Unbundle By Name(w363) -> ("C.E."=w362:refnum<class "Control Experiment.lvclass">)
        n139 = call <userlib>:"Max_Min_conversion.vi"("Min"="Vmin (start)", "Max"="Vmax (end)") -> ("offset"=w368:dbl, "Amplitude"=w367:dbl)  [unwired: 8 in]
        n140 = local read "Sweep"() -> (w352:enum16{"Vsg", "Vbg", "Z-height", ""})
        n141 = local read "Input"() -> (w355:i32[])
        n142 = call <userlib>:"Ramp.vi"("phase"="phase", "function (ramp)"="function (ramp)", "cycles (1,2,...)"="cycles (1,2,...)", "step size"="dV", "offset"=w368, "amplitude"=w367) -> ("Waveform Graph"=w364:dbl[])  [unwired: 3 in, 2 out]
        n143 = Format Into String(error in=w360, w352) -> (resulting string=w358:string, error out=w359:errorcluster)  [unwired: 2 in]
        n144 = call <userlib>:"Write Dictionary Element.vi"("error in (no error)"=w359, "value"=w364, "key"=w358, "Control Experiment in"=w362) -> ("error out"=w354:errorcluster, "Control Experiment out"=w357:refnum<class "Control Experiment.lvclass">)  [unwired: 6 in]
        n145 = case shown="\"Vsg\", Default" w352 {
          tunnel: w357 -> [w377 w383]
          tunnel: [w377 w382] -> w356
          tunnel: w355 -> [_ w381]
          tunnel: w354 -> [w376 w379]
          tunnel: [w376 w378] -> w353
          frame "Vbg" {
          }
          frame "Vsg", Default {
            n146 = call <userlib>:"Write Dictionary Element.vi"("error in (no error)"=w379, "value"=w381, "key"="Sweep Channels", "Control Experiment in"=w383) -> ("error out"=w378:errorcluster, "Control Experiment out"=w382:refnum<class "Control Experiment.lvclass">)  [unwired: 6 in]
          }
        }
        n147 = Array Size(array=w364) -> (size(s)=w361:i32)
        n148 = Bundle By Name(cluster=w363, "Sweep Values"=w364, "size"=w361, "C.E."=w356) -> (w366:T5)
        n149 = call <vilib>:"Add State(s) to Queue__jki_lib_state_machine.vi"("State(s) in (\"\")"=w375) -> ("States Out"=w374:string)  [unwired: 14 in]
      }
      frame "---------- Configure ----------" {
        # "Do not put any code in this frame.\n(It is a separator no-op. You can make a copy of this frame to create a new Macro frame)"
        n150 = call <vilib>:"Add State(s) to Queue__jki_lib_state_machine.vi"("State(s) in (\"\")"=w387) -> ("States Out"=w386:string)  [unwired: 14 in]
      }
      frame "Configure: Wait" {
        # "Do not put any code in this frame.\n(It is a separator no-op. You can make a copy of this frame to create a new Macro frame)"
        n151 = Unbundle By Name(w390) -> ("index"=w389:i32)
        n152 = case shown="Default" w389 {
          tunnel: ["Initial wait (ms)" "wait after setting Control (ms)"] -> w388
          frame 0 {
          }
          frame Default {
          }
        }
        n153 = call <userlib>:"Wait (ms)__ogtk.vi"("error in (no error)"=w392, "milliseconds to wait"=w388) -> ("error out"=w391:errorcluster)  [unwired: 8 in, 1 out]
        n154 = call <vilib>:"Add State(s) to Queue__jki_lib_state_machine.vi"("State(s) in (\"\")"=w394) -> ("States Out"=w393:string)  [unwired: 14 in]
      }
      frame "Configure: Set" {
        # "Do not put any code in this frame.\n(It is a separator no-op. You can make a copy of this frame to create a new Macro frame)"
        n155 = Unbundle By Name(w398) -> ("Instruments.Lockin"=w406:refnum<class "Instrument.Lockin.lvclass">, "Sweep Values"=w405:dbl[], "index"=w404:i32)
        n156 = Index Array(array=w405, index=w404) -> (element=w400:dbl)
        n157 = case shown="\"Z-height\"" "Sweep" {
          tunnel: w406 -> [w412 w446 w459]
          tunnel: w401 -> [w417 w445 w458]
          tunnel: w400 -> [w414 w442 w452]
          tunnel: [w416 w443 w455] -> w402
          tunnel: [w410 w441 w459] -> w397
          frame "Vsg", Default {
            n158 = call <userlib>:"getAO.vi"("Instrument.Lockin in"=w412) -> ("AOconfig"=w415:T9)  [unwired: 8 in, 2 out]
            n159 = Decrement(x="Input") -> (x-1=w411:i32[])
            n160 = for {
              tunnel: w414 -> [w439]
              shift-right: [w435] -> w409
              shift-left: w415 -> [w437]
              tunnel: w411 -> [w436] mode=indexing
              n161 = Index Array(array=w437, index=w436) -> (element=w440:T10)
              n162 = Bundle By Name(cluster=w440, "Offset"=w439) -> (w438:T10)
              n163 = Replace Array Subset(array=w437, new element=w438, index=w436) -> (w435:T9)
            }
            n164 = disable-structure shown="Enabled" {
              disable-tunnel: w417 -> [w423 w431]
              disable-tunnel: [w422 w430] -> w416
              disable-tunnel: w414 -> [w421 _]
              disable-tunnel: "Input" -> [w420 _]
              disable-tunnel: w412 -> [w419 w433]
              disable-tunnel: [w418 w432] -> w410
              disable-tunnel: w409 -> [_ w434]
              frame Disabled {
                n165 = for {
                  tunnel: w420 -> [w425] mode=indexing
                  tunnel: w421 -> [w424]
                  tunnel: w423 -> [w428]
                  tunnel: [w427] -> w422
                  shift-right: [w426] -> w418
                  shift-left: w419 -> [w429]
                  n166 = call <userlib>:"setAO_DC.vi"("error in (no error)"=w428, "DC (V)"=w424, "AO Channel"=w425, "Instrument.Lockin in"=w429) -> ("error out"=w427:errorcluster, "Instrument.Lockin out"=w426:refnum<class "Instrument.Lockin.lvclass">)  [unwired: 6 in]
                }
              }
              frame Enabled {
                n167 = call <userlib>:"setAO.vi"("error in (no error)"=w431, "Channels: AO"=w434, "Instrument.Lockin in"=w433) -> ("error out"=w430:errorcluster, "Instrument.Lockin out"=w432:refnum<class "Instrument.Lockin.lvclass">)  [unwired: 7 in]
              }
            }
          }
          frame "Vbg" {
            n168 = call <userlib>:"setAUX.vi"("error in (no error)"=w445, "AUX (V)"=w442, "Channel"=1, "Instrument.Lockin in"=w446) -> ("error out"=w443:errorcluster, "Instrument.Lockin out"=w441:refnum<class "Instrument.Lockin.lvclass">)  [unwired: 6 in]
          }
          frame "Z-height" {
            n169 = Number To Fractional String(number=w452, precision (6)=i16 7) -> (F-format string=w449:string)  [unwired: 2 in]
            n170 = call <vilib>:"Asylum_OpenRefnum.vi"("error in (no error)"=w458) -> ("error out"=w457:errorcluster, "Application"=w454:refnum<k7>)  [unwired: 9 in]
            n171 = Format Into String(format string="%s)" ("string"), initial string="td_WriteValue(\"A%Output\"," ("string"), w449) -> (resulting string=w447:string)  [unwired: 1 in, 1 out]
            n172 = call <vilib>:"Asylum_SendIgorCommand.vi"("error in (no error)"=w457, "command"=w447, "Application"=w454) -> ("error out"=w456:errorcluster, "Application"=w453:refnum<k7>)  [unwired: 5 in, 2 out]
            n173 = call <vilib>:"Asylum_CloseRefnum.vi"("error in (no error)"=w456, "Application"=w453) -> ("error out"=w455:errorcluster)  [unwired: 9 in]
          }
        }
        n174 = Bundle By Name(cluster=w398, "Instruments.Lockin"=w397) -> (w399:T5)
        n175 = call <vilib>:"Add State(s) to Queue__jki_lib_state_machine.vi"("State(s) in (\"\")"=w408) -> ("States Out"=w407:string)  [unwired: 14 in]
      }
      frame "---------- Measure ----------" {
        # "Template Separator\n(You can make a copy of, or modify, this frame)"
        n176 = call <vilib>:"Add State(s) to Queue__jki_lib_state_machine.vi"("State(s) in (\"\")"=w463) -> ("States Out"=w462:string)  [unwired: 14 in]
      }
      frame "Measure: Temperature" {
        # "Your code here.\n(You can make a copy of, or modify, this frame)"
        n177 = Unbundle By Name(w472) -> ("C.E."=w467:refnum<class "Control Experiment.lvclass">, "Instruments.Temperature"=w474:refnum<class "Instrument.Cryostat.lvclass">)
        n178 = call-dynamic "Get Temperature.vi"("error in (no error)"=w473, "Instrument.Cryostat in"=w474) -> ("error out"=w469:errorcluster, "Temperature (K)"=w465:dbl, "Instrument.Cryostat out"=w464:refnum<class "Instrument.Cryostat.lvclass">)  [unwired: 5 in, 2 out]
        "T (mK)" <- w465
        n179 = call <userlib>:"Write Dictionary Element.vi"("error in (no error)"=w469, "value"=w465, "key"="Temperature", "Control Experiment in"=w467) -> ("error out"=w468:errorcluster, "Control Experiment out"=w466:refnum<class "Control Experiment.lvclass">)  [unwired: 6 in]
        n180 = Bundle By Name(cluster=w472, "Instruments.Temperature"=w464, "C.E."=w466) -> (w471:T5)
        n181 = call <vilib>:"Add State(s) to Queue__jki_lib_state_machine.vi"("State(s) in (\"\")"=w476) -> ("States Out"=w475:string)  [unwired: 14 in]
      }
      frame "Measure: Magnet" {
        # "Your code here.\n(You can make a copy of, or modify, this frame)"
        n182 = Unbundle By Name(w486) -> ("C.E."=w482:refnum<class "Control Experiment.lvclass">, "Instruments.Magnet"=w487:refnum<class "Instrument.Cryostat.lvclass">)
        n183 = call-dynamic "Get Magnet.vi"("error in (no error)"=w484, "Instrument.Cryostat in"=w487) -> ("error out"=w479:errorcluster, "B Field (T)"=w481:dbl, "Instrument.Cryostat out"=w478:refnum<class "Instrument.Cryostat.lvclass">)  [unwired: 5 in, 2 out]
        "Field (T)" <- w481
        n184 = call <userlib>:"Write Dictionary Element.vi"("error in (no error)"=w479, "value"=w481, "key"="Magnet", "Control Experiment in"=w482) -> ("error out"=w480:errorcluster, "Control Experiment out"=w483:refnum<class "Control Experiment.lvclass">)  [unwired: 6 in]
        n185 = Bundle By Name(cluster=w486, "Instruments.Magnet"=w478, "C.E."=w483) -> (w485:T5)
        n186 = call <vilib>:"Add State(s) to Queue__jki_lib_state_machine.vi"("State(s) in (\"\")"=w489) -> ("States Out"=w488:string)  [unwired: 14 in]
      }
      frame "Measure: Capacitance" {
        # "Your code here.\n(You can make a copy of, or modify, this frame)"
        n187 = Unbundle By Name(w497) -> ("C.E."=w498:refnum<class "Control Experiment.lvclass">, "Instruments.Capacitance Bridge"=w500:refnum<class "Instrument.CBridge.lvclass">)
        n188 = call-dynamic "Get Capacitance.vi"("error in (no error)"=w494, "Instrument.CBridge in"=w500) -> ("error out"=w499:errorcluster, "Capacitance (pF)"=w490:dbl, "Instrument.CBridge out"=w491:refnum<class "Instrument.CBridge.lvclass">)  [unwired: 7 in]
        n189 = call <userlib>:"Write Dictionary Element.vi"("error in (no error)"=w499, "value"=w490, "key"="Capacitance", "Control Experiment in"=w498) -> ("error out"=w493:errorcluster, "Control Experiment out"=w495:refnum<class "Control Experiment.lvclass">)  [unwired: 6 in]
        n190 = Bundle By Name(cluster=w497, "Instruments.Capacitance Bridge"=w491, "C.E."=w495) -> (w496:T5)
        n191 = call <vilib>:"Add State(s) to Queue__jki_lib_state_machine.vi"("State(s) in (\"\")"=w502) -> ("States Out"=w501:string)  [unwired: 14 in]
      }
      frame "Measure: Lockin" {
        # "Template Separator\n(You can make a copy of, or modify, this frame)"
        n192 = Unbundle By Name(w515) -> ("C.E."=w514:refnum<class "Control Experiment.lvclass">, "Instruments.Lockin"=w517:refnum<class "Instrument.Lockin.lvclass">)
        n193 = call <userlib>:"waitForNewResults.vi"("error in (no error)"=w518, "Instrument.Lockin in"=w517) -> ("error out"=w512:errorcluster, "Results (Dictionary)"=w506:cluster{"key":string, "value":dbl}[], "Instrument.Lockin out"=w510:refnum<class "Instrument.Lockin.lvclass">)  [unwired: 7 in]
        n194 = call <userlib>:"Parse Results (all).vi"("Type"=Results_Type--Enum."Y", "Results (Dictionary)"=w506) -> ("Data"=w504:dbl[])  [unwired: 6 in, 3 out]
        n195 = call <userlib>:"Parse Results (all).vi"("Type"=Results_Type--Enum."Mean", "Results (Dictionary)"=w506) -> ("Data"=w503:dbl[])  [unwired: 6 in, 3 out]
        n196 = call <userlib>:"Parse Results (all).vi"("Type"=Results_Type--Enum."X", "Results (Dictionary)"=w506) -> ("Data"=w508:dbl[])  [unwired: 6 in, 3 out]
        n197 = for {
          tunnel: w508 -> [w536] mode=indexing
          tunnel: w504 -> [w531] mode=indexing
          tunnel: w512 -> [w530]
          tunnel: [w527] -> w511
          shift-right: [w528] -> w513
          shift-left: w514 -> [w539]
          tunnel: w503 -> [w523] mode=indexing
          i -> [w542]
          n198 = Increment(x=w542) -> (x+1=w526:i32)
          n199 = Format Into String(format string="X%d" ("wavenames"), error in=w530, w526) -> (resulting string=w538:string, error out=w534:errorcluster)  [unwired: 1 in]
          n200 = call <userlib>:"Append Dictionary Element.vi"("error in (no error)"=w534, "value"=w536, "key"=w538, "Control Experiment in"=w539) -> ("error out"=w533:errorcluster, "Control Experiment out"=w535:refnum<class "Control Experiment.lvclass">)  [unwired: 6 in]
          n201 = Format Into String(format string="Y%d" ("wavenames"), error in=w533, w526) -> (resulting string=w537:string, error out=w532:errorcluster)  [unwired: 1 in]
          n202 = call <userlib>:"Append Dictionary Element.vi"("error in (no error)"=w532, "value"=w531, "key"=w537, "Control Experiment in"=w535) -> ("error out"=w522:errorcluster, "Control Experiment out"=w529:refnum<class "Control Experiment.lvclass">)  [unwired: 6 in]
          n203 = Format Into String(format string="Mean%d" ("wavenames"), error in=w522, w526) -> (resulting string=w524:string, error out=w521:errorcluster)  [unwired: 1 in]
          n204 = call <userlib>:"Append Dictionary Element.vi"("error in (no error)"=w521, "value"=w523, "key"=w524, "Control Experiment in"=w529) -> ("error out"=w527:errorcluster, "Control Experiment out"=w528:refnum<class "Control Experiment.lvclass">)  [unwired: 6 in]
        }
        n205 = Bundle By Name(cluster=w515, "Instruments.Lockin"=w510, "Results (Dictionary)"=w506, "C.E."=w513) -> (w516:T5)
        n206 = call <vilib>:"Add State(s) to Queue__jki_lib_state_machine.vi"("State(s) in (\"\")"=w520) -> ("States Out"=w519:string)  [unwired: 14 in]
      }
      frame "Measure: Time" {
        # "Your code here.\n(You can make a copy of, or modify, this frame)"
        n207 = Unbundle By Name(w549) -> ("C.E."=w548:refnum<class "Control Experiment.lvclass">)
        n208 = Get Date/Time In Seconds() -> (seconds since 1Jan1904=w551:timestamp)
        n209 = To Double Precision Float(number=w551) -> (double precision float=w546:dbl)
        n210 = call <userlib>:"Write Dictionary Element.vi"("error in (no error)"=w545, "value"=w546, "key"="Time", "Control Experiment in"=w548) -> ("error out"=w544:errorcluster, "Control Experiment out"=w547:refnum<class "Control Experiment.lvclass">)  [unwired: 6 in]
        n211 = Bundle By Name(cluster=w549, "C.E."=w547) -> (w550:T5)
        n212 = call <vilib>:"Add State(s) to Queue__jki_lib_state_machine.vi"("State(s) in (\"\")"=w553) -> ("States Out"=w552:string)  [unwired: 14 in]
      }
      frame "---------- File ----------" {
        # "Template Separator\n(You can make a copy of, or modify, this frame)"
        n213 = call <vilib>:"Add State(s) to Queue__jki_lib_state_machine.vi"("State(s) in (\"\")"=w557) -> ("States Out"=w556:string)  [unwired: 14 in]
      }
      frame "File: Configure" {
        # "Template Separator\n(You can make a copy of, or modify, this frame)"
        n214 = call <vilib>:"Add State(s) to Queue__jki_lib_state_machine.vi"("State(s) in (\"\")"=w561) -> ("States Out"=w560:string)  [unwired: 14 in]
      }
      frame "File: Save" {
        # "Template Separator\n(You can make a copy of, or modify, this frame)"
        n215 = Unbundle By Name(w564) -> ("C.E."=w569:refnum<class "Control Experiment.lvclass">, "Execution:State"=w566:T6)
        n216 = call <userlib>:"Exec State to Append.vi"("Execution:State"=w566) -> ("append?"=w565:bool)  [unwired: 2 in]
        n217 = call <userlib>:"Save Transport TDMS File.vi"("error in (no error)"=w567, "append?"=w565, "Control Experiment in"=w569) -> ("error out"=w568:errorcluster, "Control Experiment out"=w562:refnum<class "Control Experiment.lvclass">)  [unwired: 7 in]
        n218 = Bundle By Name(cluster=w564, "C.E."=w562) -> (w563:T5)
        n219 = call <vilib>:"Add State(s) to Queue__jki_lib_state_machine.vi"("State(s) in (\"\")"=w571) -> ("States Out"=w570:string)  [unwired: 14 in]
      }
    }
  }
  "error out" <- w2
  n220 = Unbundle By Name(w4) -> ("Transport"=→"Transport.lvclass":refnum<class "Transport.lvclass">)
